vi "PIM Check for Matching Channel.vi"(9 "Match Channels":T1[](array[typedef]), 10 "Channel Name":string) -> (2 "Match Found?":bool)   [LabVIEW 2011]
uses:
  TypeDefs/PIM Data Channels.ctl
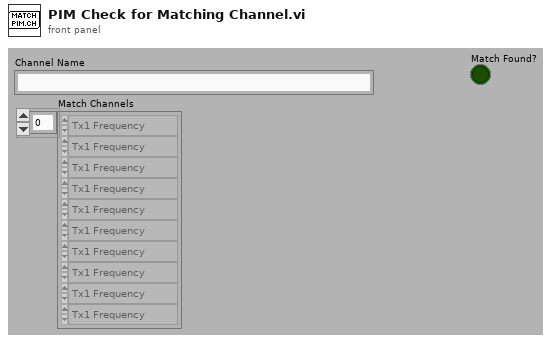
[diagram p1: front panel]
types:
  T1 = typedef "PIM Data Channels.ctl" = enum16{"Tx1 Frequency", "Tx1 Power", "Tx1 Check Tx", "Tx1 Unleveled", "Tx1 Squelch", "Tx2 Frequency", "Tx2 Power", "Tx2 Check Tx", "Tx2 Unleveled", "Tx2 Squelch", "Elapsed Time", "Ref Limit 1", "Ref Limit 2", "IM Overload", "IM%d Frequency", "IM%d Power 1", "IM%d Power 2"}
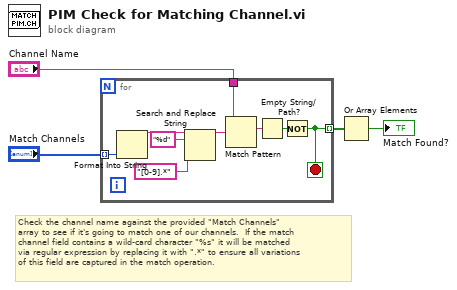
[diagram p0: block diagram]
diagram:
  # "Check the channel name against the provided \"Match Channels\"\narray to see if it's going to match one of our channels.  If the match\nchannel field contains a wild-card character \"%s\" it will be matched\nvia regular expression by replacing it with \".*\" to ensure all variations\nof this field are captured in the match operation."
  n1 = for {
    tunnel: "Channel Name" -> [w9]
    tunnel: [w5] -> w3 mode=indexing
    tunnel: "Match Channels" -> [w6] mode=indexing
    stop <- w5 stop-if-true
    n2 = Format Into String(w6) -> (resulting string=w13:string)  [unwired: 3 in, 1 out]
    n3 = Search and Replace String(input string=w13, search string="%d", replace string="[0-9].*" ("replace string (\"\")")) -> (result string=w10:string)  [unwired: 1 in, 7 out]
    n4 = Match Pattern(string=w9, regular expression=w10) -> (match substring=w8:string)  [unwired: 4 out]
    n5 = Empty String/Path?(string/path=w8) -> (empty?=w7:bool)
    n6 = Not(x=w7) -> (.not. x?=w5:bool)
  }
  n7 = Or Array Elements(Boolean array=w3) -> (logical OR=→"Match Found?":bool)
